vi "prediction bounds.vi"(6 "damping":dbl, 7 "amplitude":dbl, 8 "error in (no error)":errorcluster, 9 "Hours array":dbl[](array[numeric]), 10 "Previous Hours Array":dbl[](array[numeric]), 11 "Previous Data Array":dbl[](array[numeric])) -> (0 "error out":errorcluster, 1 "Lower Bound":cluster{dbl, "p(x)":dbl}[](array[cluster]), 3 "Upper Bound":cluster{dbl, "p(x)":dbl}[](array[cluster]))   [LabVIEW 2013]
uses:
  <vilib>/Analysis/6fits.llb/Prediction Interval (Exp).vi
  <vilib>/Analysis/polynomials.llb/1D Polynomial Evaluation (DBL).vi
  <vilib>/Analysis/NI_AALPro.lvlib
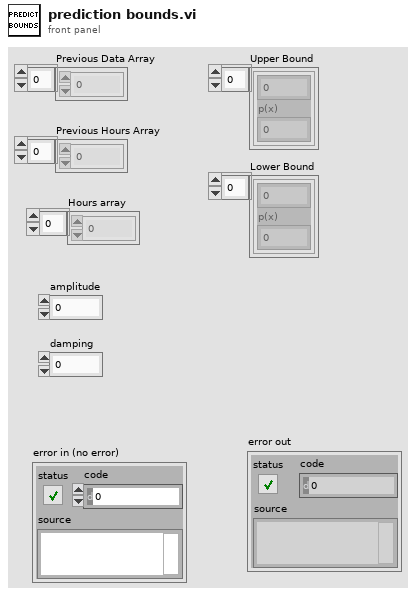
[diagram p1: front panel]
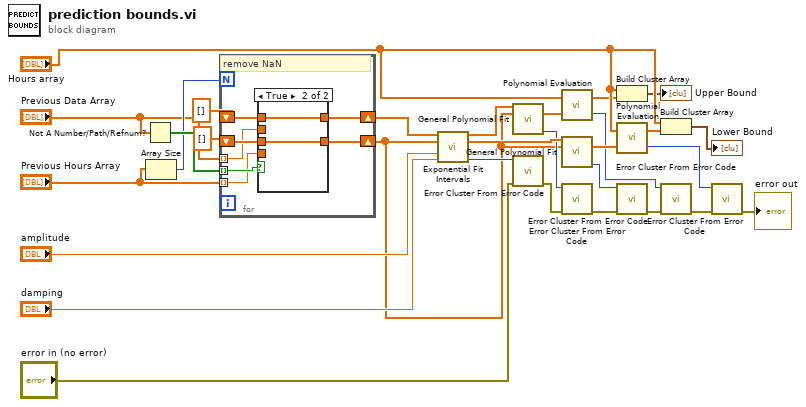
[diagram p0: block diagram]
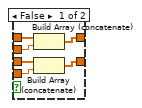
[diagram p2: hidden frame]
diagram:
  n1 = Not A Number/Path/Refnum?(number/path/refnum="Previous Data Array") -> (NaN/Path/Refnum?=w8:bool[])
  n2 = Array Size(array="Previous Hours Array") -> (size(s)=w7:i32)
  n3 = for {
    N: w7 -> [_]
    tunnel: w8 -> [w37] mode=indexing
    shift-right: [w36] -> w1
    shift-left: dbl[] [] -> [w35]
    shift-right: [w34] -> w4
    shift-left: dbl[] [] -> [w33]
    tunnel: "Previous Hours Array" -> [w32] mode=indexing
    tunnel: "Previous Data Array" -> [w31] mode=indexing
    # "remove NaN"
    n4 = case shown="True" w37 {
      tunnel: [w42 w45] -> w36
      tunnel: w35 -> [w43 w45]
      tunnel: [w41 w44] -> w34
      tunnel: w33 -> [w40 w44]
      tunnel: w32 -> [w39 _]
      tunnel: w31 -> [w38 _]
      frame False {
        n5 = Build Array (concatenate)(w40, w38) -> (w41:dbl[])
        n6 = Build Array (concatenate)(w43, w39) -> (w42:dbl[])
      }
      frame True {
      }
    }
  }
  n7 = call-poly <vilib>:"Exponential Fit Intervals.vi"("Y"=w4, "X"=w1, "amplitude"="amplitude", "damping"="damping") -> ("Upper Bound"=w25:dbl[], "Lower Bound"=w22:dbl[], "error"=w19:i32)  [unwired: 9 in]
  n8 = call <vilib>:"General Polynomial Fit.vi"("Y"=w25, "X"=w1) -> ("Polynomial Coefficients"=w27:dbl[], "error"=w14:i32)  [unwired: 10 in, 2 out]
  n9 = call <vilib>:"Error Cluster From Error Code.vi"("error in (no error)"="error in (no error)", "error code (0)"=w19) -> ("error out"=w17:errorcluster)  [unwired: 7 in]
  n10 = call-poly <vilib>:"Polynomial Evaluation.vi"("P(x)"=w27, "A"="Hours array") -> ("error"=w12:i32, "P(A)"=w28:dbl[])
  n11 = call <vilib>:"General Polynomial Fit.vi"("Y"=w22, "X"=w1) -> ("Polynomial Coefficients"=w24:dbl[], "error"=w13:i32)  [unwired: 10 in, 2 out]
  n12 = call <vilib>:"Error Cluster From Error Code.vi"("error in (no error)"=w17, "error code (0)"=w14) -> ("error out"=w16:errorcluster)  [unwired: 7 in]
  n13 = Build Cluster Array("Hours array", w28) -> (→"Upper Bound":cluster{dbl, "p(x)":dbl}[])
  n14 = call-poly <vilib>:"Polynomial Evaluation.vi"("P(x)"=w24, "A"="Hours array") -> ("error"=w10:i32, "P(A)"=w23:dbl[])
  n15 = call <vilib>:"Error Cluster From Error Code.vi"("error in (no error)"=w16, "error code (0)"=w13) -> ("error out"=w15:errorcluster)  [unwired: 7 in]
  n16 = Build Cluster Array("Hours array", w23) -> (→"Lower Bound":cluster{dbl, "p(x)":dbl}[])
  n17 = call <vilib>:"Error Cluster From Error Code.vi"("error in (no error)"=w15, "error code (0)"=w12) -> ("error out"=w11:errorcluster)  [unwired: 7 in]
  n18 = call <vilib>:"Error Cluster From Error Code.vi"("error in (no error)"=w11, "error code (0)"=w10) -> ("error out"=→"error out":errorcluster)  [unwired: 7 in]
